vi "Read Messages.vi"(8 "error in":errorcluster, 11 "port in":T1 format="%.0x") -> (0 "error out":errorcluster, 2 "messages":T2[](array[typedef]), 3 "port out":T1 format="%.0x")   [LabVIEW 2020, in "Ballard MIL-STD-1553 Scripting.lvlib"]
uses:
  Ballard MIL-STD-1553 Scripting.lvlib
  Shared/Message Definition.ctl
  Shared/Message Type.ctl
  Shared/Terminal Endpoint.ctl
  Shared/Address.ctl
  Shared/Parameter Definition.ctl
  <vilib>/NI VeriStand/Custom Device API/Custom Device Item Ref.ctl
  <vilib>/NI VeriStand/Custom Device API/Custom Device API.lvlib
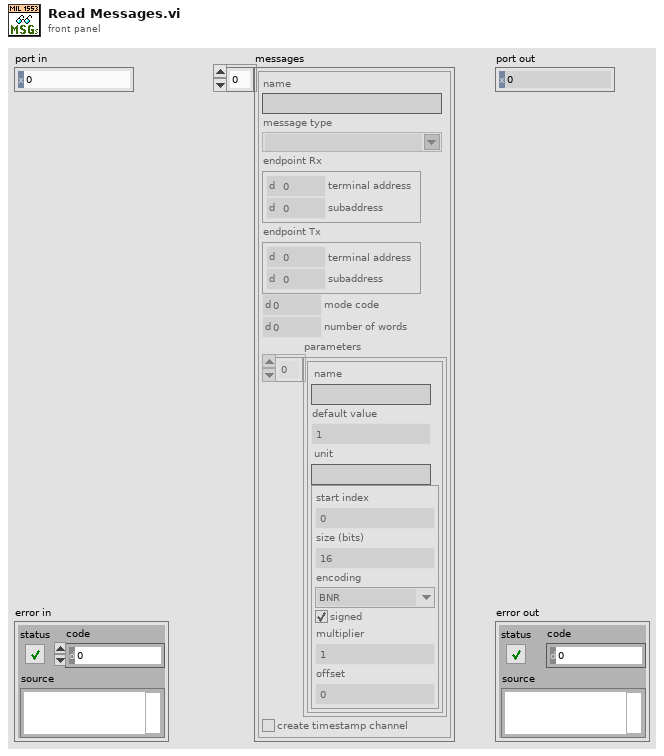
[diagram p1: front panel]
types:
  T1 = typedef "Custom Device API.lvlib/Custom Device Item Ref.ctl" = u64
  T2 = typedef "Message Definition.ctl" = cluster{"name":string, "message type":T3, "endpoint Rx":T4, "endpoint Tx":T4, "mode code":u16, "number of words":u16, "parameters":cluster{"name":string, "default value":dbl, "unit":string, "parameter definition":T6}[], "create timestamp channel":bool}
  T3 = typedef "Message Type.ctl" = string
  T4 = typedef "Terminal Endpoint.ctl" = cluster{"terminal address":T5, "subaddress":T5}
  T5 = typedef "Address.ctl" = u16
  T6 = typedef "Parameter Definition.ctl" = cluster{"start index":i32, "size (bits)":i32, "encoding":enum16{"BNR", "BCD", "Discrete"}, "signed":bool, "multiplier":dbl, "offset":dbl}
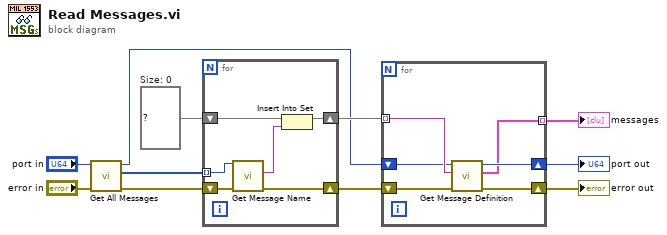
[diagram p0: block diagram]
diagram:
  w10 = set{string} {}  # Size: 0
  n1 = call "Get All Messages.vi"("error in"="error in", "port in"="port in") -> ("error out"=w8:errorcluster, "messages"=w9:T1[], "port out"=w3:T1)  [unwired: 7 in]
  n2 = for {
    shift-right: [w17] -> w5
    shift-left: w8 -> [w16]
    tunnel: w9 -> [w15] mode=indexing
    shift-right: [w13] -> w11
    shift-left: w10 -> [w12]
    n3 = call "Get Message Name.vi"("error in"=w16, "message in"=w15) -> ("error out"=w17:errorcluster, "message name"=w14:string)  [unwired: 6 in, 2 out]
    n4 = Insert Into Set(10:w14, 11:w12) -> (3:w13:set{string})  [unwired: 1 out]
  }
  n5 = for {
    tunnel: w11 -> [w22] mode=indexing
    shift-right: [w19] -> w4
    shift-left: w5 -> [w23]
    shift-right: [w20] -> w2
    shift-left: w3 -> [w21]
    tunnel: [w18] -> w1 mode=indexing
    n6 = call "Get Message Definition.vi"("error in"=w23, "message name"=w22, "port in"=w21) -> ("error out"=w19:errorcluster, "message configuration"=w18:T2, "port out"=w20:T1)  [unwired: 6 in]
  }
  "messages" <- w1
  "error out" <- w4
  "port out" <- w2
